vi "GetProperties.vi"(8 "error in (no error)":errorcluster, 9 "appKey":string, 10 "url beginning":string, 11 "client handle":T1) -> (0 "error out":errorcluster, 1 "result string":string, 2 "Array":string[][](array[string]), 3 "client handle out":T1, 5 "ThingWorx Response":string)   [LabVIEW 2015]
uses:
  <vilib>/httpClient/ClientHandle.ctl
  <vilib>/httpClient/LabVIEWHTTPClient.lvlib
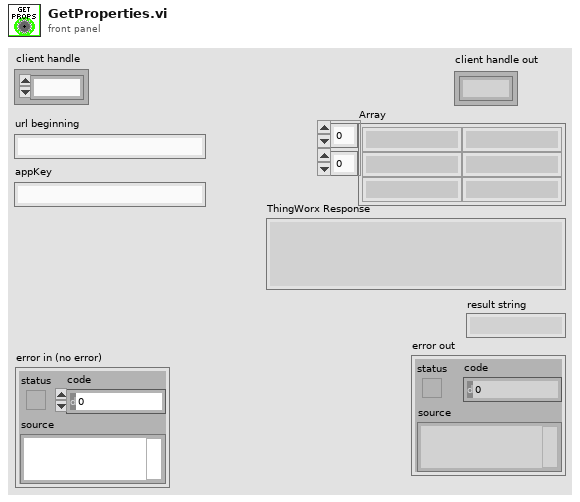
[diagram p1: front panel]
types:
  T1 = typedef "LabVIEWHTTPClient.lvlib/ClientHandle.ctl" = refnum<k1>
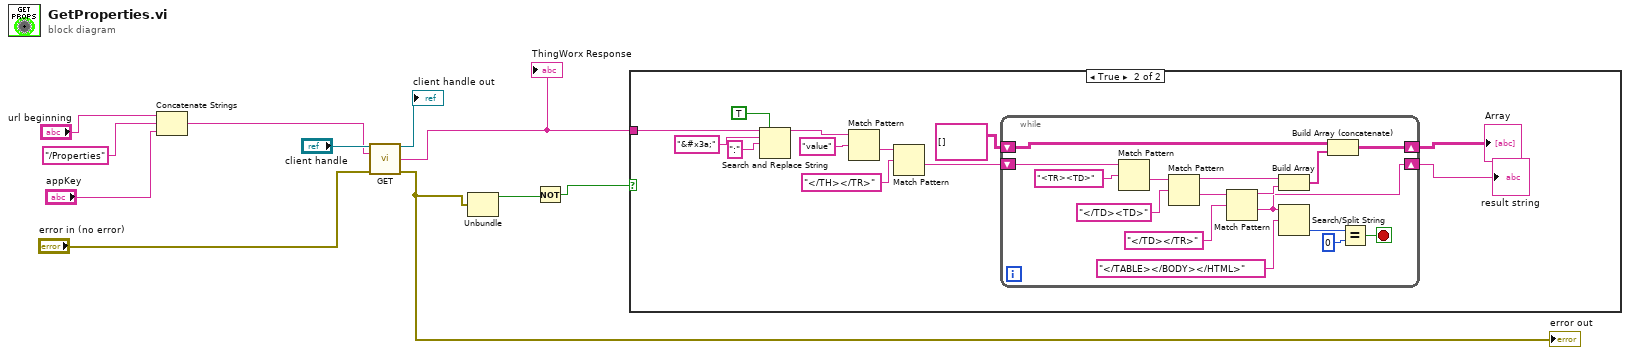
[diagram p0: block diagram]
diagram:
  n1 = Concatenate Strings("url beginning", "/Properties" ("url"), "appKey") -> (w5:string)
  n2 = call <vilib>:"GET.vi"("client handle"="client handle", "url"=w5, "error in (no error)"="error in (no error)") -> ("client handle out"=→"client handle out":T1, "body"=w11:string, "error out"=w3:errorcluster)  [unwired: 9 in, 1 out]
  "error out" <- w3
  "ThingWorx Response" <- w11
  n3 = Unbundle(w3) -> ("status"=w2:bool)  [unwired: 2 out]
  n4 = Not(x=w2) -> (.not. x?=w1:bool)
  n5 = case shown="True" w1 {
    tunnel: w11 -> [_ w12]
    frame False {
    }
    frame True {
      n6 = Search and Replace String(replace all?=TRUE ("replace all? (F)"), input string=w12, search string="&#x3a;", replace string=":" ("replace string (\"\")")) -> (result string=w21:string)  [unwired: 4 in, 3 out]
      n7 = Match Pattern(string=w21, regular expression="value") -> (after substring=w15:string)  [unwired: 1 in, 3 out]
      n8 = Match Pattern(string=w15, regular expression="</TH></TR>") -> (after substring=w17:string)  [unwired: 1 in, 3 out]
      n9 = while {
        shift-right: [w28] -> w19
        shift-left: w17 -> [w25]
        shift-right: [w29] -> w18
        shift-left: string[][] [] -> [w39]
        stop <- w27 stop-if-true
        n10 = Match Pattern(string=w25, regular expression="<TR><TD>") -> (after substring=w24:string)  [unwired: 1 in, 3 out]
        n11 = Match Pattern(string=w24, regular expression="</TD><TD>") -> (before substring=w37:string, after substring=w31:string)  [unwired: 1 in, 2 out]
        n12 = Match Pattern(string=w31, regular expression="</TD></TR>") -> (before substring=w30:string, after substring=w28:string)  [unwired: 1 in, 2 out]
        n13 = Build Array(w37, w30) -> (w36:string[])
        n14 = Search/Split String(string=w28, search string/char (-)="</TABLE></BODY></HTML>" ("true string")) -> (offset of match=w34:i32)  [unwired: 1 in, 2 out]
        n15 = Build Array (concatenate)(w39, w36) -> (w29:string[][])
        n16 = Equal?(x=w34, y=0) -> (x = y?=w27:bool)
      }
      "result string" <- w19
      "Array" <- w18
    }
  }
